vi "First Level.vi"() -> (0 "2D Picture":picture)   [LabVIEW 2014]
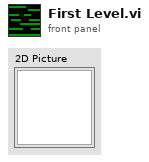
[diagram p1: front panel]
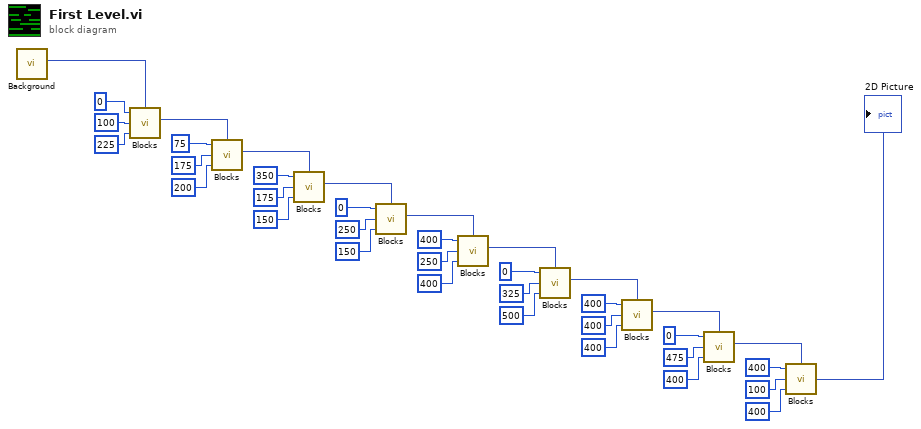
[diagram p0: block diagram]
diagram:
  n1 = call "Background.vi"() -> (w7:picture)
  n2 = call "Blocks.vi"("Input Picture"=w7, "Width"=i16 225, "Origin Y"=i16 100, "Origin X"=i16 0) -> (0:w11:picture)
  n3 = call "Blocks.vi"("Input Picture"=w11, "Width"=i16 200, "Origin Y"=i16 175, "Origin X"=i16 75) -> (0:w18:picture)
  n4 = call "Blocks.vi"("Input Picture"=w18, "Width"=i16 150, "Origin Y"=i16 175, "Origin X"=i16 350) -> (0:w19:picture)
  n5 = call "Blocks.vi"("Input Picture"=w19, "Width"=i16 150, "Origin Y"=i16 250, "Origin X"=i16 0) -> (0:w20:picture)
  n6 = call "Blocks.vi"("Input Picture"=w20, "Width"=i16 400, "Origin Y"=i16 250, "Origin X"=i16 400) -> (0:w24:picture)
  n7 = call "Blocks.vi"("Input Picture"=w24, "Width"=i16 500, "Origin Y"=i16 325, "Origin X"=i16 0) -> (0:w28:picture)
  n8 = call "Blocks.vi"("Input Picture"=w28, "Width"=i16 400, "Origin Y"=i16 400, "Origin X"=i16 400) -> (0:w32:picture)
  n9 = call "Blocks.vi"("Input Picture"=w32, "Width"=i16 400, "Origin Y"=i16 475, "Origin X"=i16 0) -> (0:w36:picture)
  n10 = call "Blocks.vi"("Input Picture"=w36, "Width"=i16 400, "Origin Y"=i16 100, "Origin X"=i16 400) -> (0:→"2D Picture":picture)
